vi "test Add-Find-Remove Subaddress.vi"(8 "error in":errorcluster, 11 "TestCase in":refnum<class "Scripting.lvclass">) -> (0 "error out":errorcluster, 3 "TestCase out":refnum<class "Scripting.lvclass">)   [LabVIEW 2020, in "Scripting.lvclass"]
uses:
  Scripting.lvclass
  <vilib>/addons/_JKI Toolkits/VI Tester/TestCase.llb/TestCase.lvclass
  Scripting/AIM MIL-STD-1553 Scripting.lvlib
  Shared/Address.ctl
  C:/Program Files (x86)/National Instruments/LabVIEW 2020/vi.lib/NI/VeriStand Custom Device Testing Tools/VeriStandScriptingTestCase/VeriStandScriptingTestCase.lvclass
  C:/Program Files (x86)/National Instruments/LabVIEW 2020/vi.lib/addons/_JKI Toolkits/VI Tester/TestCase.llb/TestCase.lvclass
  C:/Users/nitest/Desktop/Git/niveristand-aim-milStd1553-custom-device/Source/Custom Device Support/Tests/Unit/Scripting/Scripting.lvclass
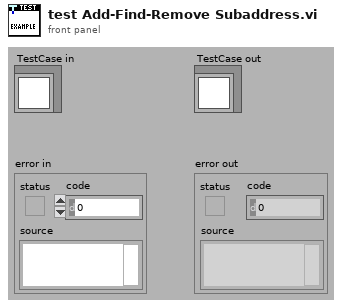
[diagram p1: front panel]
types:
  T1 = typedef "Address.ctl" = u16
  T2 = typedef "Custom Device API.lvlib/Custom Device Item Ref.ctl" = u64
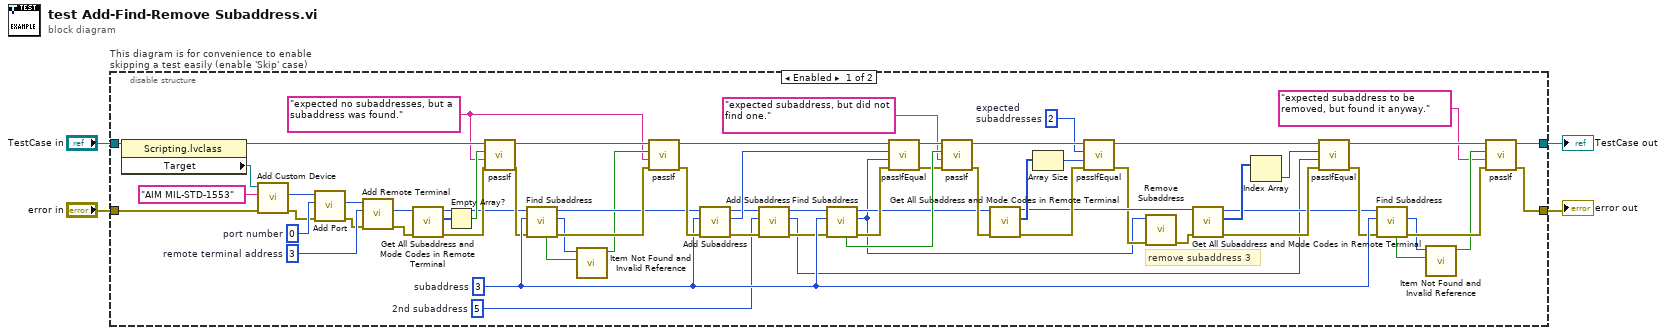
[diagram p0: block diagram]
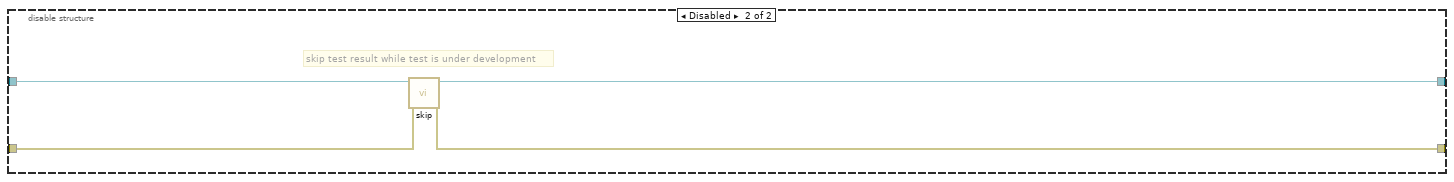
[diagram p2: hidden frame]
diagram:
  n1 = disable-structure "This diagram is for convenience to enable skipping a test easily (enable 'Skip' case)" shown="Enabled" {
    disable-tunnel: "TestCase in" -> [w67 w73]
    disable-tunnel: [w62 w71] -> w1
    disable-tunnel: [w63 w72] -> w3
    disable-tunnel: "error in" -> [w69 w70]
    frame Enabled {
      w13 = "expected no subaddresses, but a subaddress was found." ("message (\"\")")
      w21 = T1 3  # remote terminal address
      w32 = 2  # expected  subaddresses
      w39 = T1 5  # 2nd subaddress
      w53 = T1 3  # subaddress
      w65 = u16 0  # port number
      # "remove subaddress 3"
      n2 = property class="Scripting.lvclass"(reference=w67) -> (reference out=w50:refnum<class "Scripting.lvclass">, "Target"=w66:refnum<k24>)  [unwired: 1 in, 1 out]
      n3 = call "Add Custom Device.vi"("error in"=w69, "custom device name"="AIM MIL-STD-1553" ("name"), "target"=w66) -> ("error out"=w47:errorcluster, "custom device"=w48:T2)  [unwired: 6 in, 1 out]
      n4 = call "Add Port.vi"("error in"=w47, "port number"=w65, "custom device"=w48) -> ("error out"=w20:errorcluster, "port"=w22:T2)  [unwired: 6 in, 1 out]
      n5 = call "Add Remote Terminal.vi"("error in"=w20, "terminal address"=w21, "port"=w22) -> ("error out"=w19:errorcluster, "remote terminal"=w18:T2)  [unwired: 6 in, 1 out]
      n6 = call "Get All Subaddress and Mode Codes in Remote Terminal.vi"("error in"=w19, "remote terminal"=w18) -> ("error out"=w46:errorcluster, "subaddress sections"=w51:T2[], "remote terminal out"=w44:T2)  [unwired: 7 in]
      n7 = Empty Array?(array=w51) -> (empty?=w52:bool)
      n8 = call-dynamic "passIf.vi"("error in (no error)"=w46, "message (\"\")"=w13, "pass"=w52, "TestCase in"=w50) -> ("error out"=w45:errorcluster, "TestCase out"=w49:refnum<class "Scripting.lvclass">)  [unwired: 6 in]
      n9 = call "Find Subaddress.vi"("error in"=w45, "subaddress"=w53, "remote terminal"=w44) -> ("error out"=w60:errorcluster, "subaddress section"=w16:T2, "remote terminal out"=w30:T2, "found?"=w15:bool)  [unwired: 5 in]
      n10 = call "Item Not Found and Invalid Reference.vi"("found?"=w15, "item reference"=w16) -> ("no item found"=w14:bool)  [unwired: 9 in]
      n11 = call-dynamic "passIf.vi"("error in (no error)"=w60, "message (\"\")"=w13, "pass"=w14, "TestCase in"=w49) -> ("error out"=w61:errorcluster, "TestCase out"=w59:refnum<class "Scripting.lvclass">)  [unwired: 6 in]
      n12 = call "Add Subaddress.vi"("error in"=w61, "subaddress"=w53, "remote terminal"=w30) -> ("error out"=w40:errorcluster, "subaddress section"=w58:T2, "remote terminal out"=w41:T2)  [unwired: 6 in]
      n13 = call "Add Subaddress.vi"("error in"=w40, "subaddress"=w39, "remote terminal"=w41) -> ("error out"=w43:errorcluster, "subaddress section"=w23:T2, "remote terminal out"=w42:T2)  [unwired: 6 in]
      n14 = call "Find Subaddress.vi"("error in"=w43, "subaddress"=w53, "remote terminal"=w42) -> ("error out"=w57:errorcluster, "subaddress section"=w9:T2, "remote terminal out"=w37:T2, "found?"=w56:bool)  [unwired: 5 in]
      n15 = call-dynamic "passIfEqual.vi"("error in (no error)"=w57, "y"=w9, "x"=w58, "TestCase in"=w59) -> ("error out"=w55:errorcluster, "TestCase out"=w64:refnum<class "Scripting.lvclass">)  [unwired: 6 in]
      n16 = call-dynamic "passIf.vi"("error in (no error)"=w55, "message (\"\")"="expected subaddress, but did not find one." ("message (\"\")"), "pass"=w56, "TestCase in"=w64) -> ("error out"=w38:errorcluster, "TestCase out"=w36:refnum<class "Scripting.lvclass">)  [unwired: 6 in]
      n17 = call "Get All Subaddress and Mode Codes in Remote Terminal.vi"("error in"=w38, "remote terminal"=w37) -> ("error out"=w35:errorcluster, "subaddress sections"=w34:T2[], "remote terminal out"=w31:T2)  [unwired: 7 in]
      n18 = Array Size(array=w34) -> (size(s)=w33:i32)
      n19 = call-dynamic "passIfEqual.vi"("error in (no error)"=w35, "y"=w33, "x"=w32, "TestCase in"=w36) -> ("error out"=w10:errorcluster, "TestCase out"=w28:refnum<class "Scripting.lvclass">)  [unwired: 6 in]
      n20 = call "Remove Subaddress.vi"("error in"=w10, "remote terminal"=w9) -> ("error out"=w11:errorcluster)  [unwired: 9 in]
      n21 = call "Get All Subaddress and Mode Codes in Remote Terminal.vi"("error in"=w11, "remote terminal"=w31) -> ("error out"=w26:errorcluster, "subaddress sections"=w29:T2[], "remote terminal out"=w24:T2)  [unwired: 7 in]
      n22 = Index Array(array=w29) -> (element=w17:T2)  [unwired: 1 in]
      n23 = call-dynamic "passIfEqual.vi"("error in (no error)"=w26, "y"=w23, "x"=w17, "TestCase in"=w28) -> ("error out"=w25:errorcluster, "TestCase out"=w27:refnum<class "Scripting.lvclass">)  [unwired: 6 in]
      n24 = call "Find Subaddress.vi"("error in"=w25, "subaddress"=w53, "remote terminal"=w24) -> ("error out"=w54:errorcluster, "subaddress section"=w8:T2, "found?"=w7:bool)  [unwired: 5 in, 1 out]
      n25 = call "Item Not Found and Invalid Reference.vi"("found?"=w7, "item reference"=w8) -> ("no item found"=w6:bool)  [unwired: 9 in]
      n26 = call-dynamic "passIf.vi"("error in (no error)"=w54, "message (\"\")"="expected subaddress to be removed, but found it anyway." ("message (\"\")"), "pass"=w6, "TestCase in"=w27) -> ("error out"=w63:errorcluster, "TestCase out"=w62:refnum<class "Scripting.lvclass">)  [unwired: 6 in]
    }
    frame Disabled {
      # "skip test result while test is under development"
      n27 = call <vilib>:"skip.vi"("error in (no error)"=w70, "TestCase in"=w73) -> ("error out"=w72:errorcluster, "TestCase out"=w71:refnum<class "Scripting.lvclass">)  [unwired: 8 in]
    }
  }
  "error out" <- w3
  "TestCase out" <- w1
